vi "test.vi"() -> ()   [LabVIEW 2025]
panel:
  in  "Time Constant":dbl
  out "Output":dbl
  in  "Boolean":bool
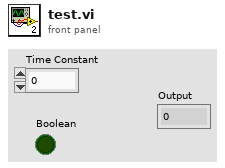
[diagram p1: front panel]
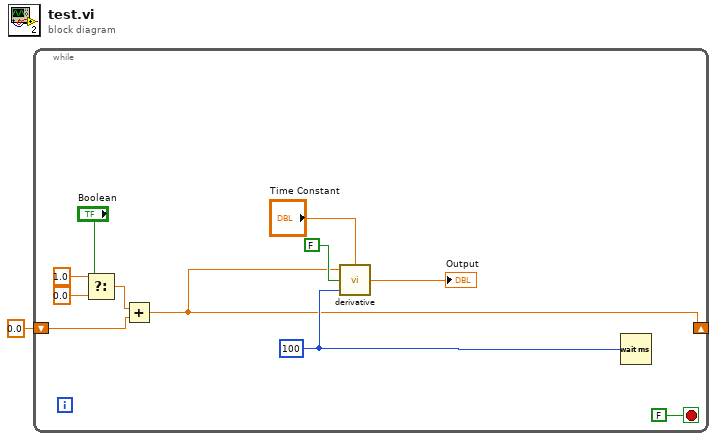
[diagram p0: block diagram]
diagram:
  n1 = while {
    shift-right: [w2] -> _
    shift-left: 0.0 -> [w7]
    stop <- FALSE stop-if-true
    w10 = u32 100 ("milliseconds to wait")
    n2 = Select(t=1.0, s="Boolean", f=0.0) -> (s? t:f=w6:dbl)
    n3 = Add(x=w6, y=w7) -> (x+y=w2:dbl)
    n4 = call "derivative.vi"("Time Constant"="Time Constant", "dt_ms"=w10, "IC"=FALSE, "Input"=w2) -> ("Output"=→"Output":dbl)
    n5 = Wait (ms)(milliseconds to wait=w10) -> ()  [unwired: 1 out]
  }
